vi "Acquisition Engine State Machine.vi"(5 "Start Next Record":bool, 7 "Record Parameters":T2={"Load Record Parameters?"=FALSE, "Pre Trigger Samples"=0, "Post Trigger Samples"=1000, "Trigger Hold Off"=0, "Record Count"=1}, 8 "Trigger Info":cluster{"Trigger":bool, "Trig Offset":u8}={"Trigger"=TRUE, "Trig Offset"=0}, 10 "Arm Acquisition Engine":bool, 11 "Input":i16[](array[numeric])=[0, 0, 0, 0, 0, 0, 0, 0]) -> (0 "Trigger Info":cluster{"Trigger":bool, "Trig Offset":u8}, 1 "PostTrigComplete":bool, 2 "AcqInProgress":bool, 3 "Output":i16[](array[numeric]), 4 "States":T1, 6 "Record Count":u32)   [LabVIEW 2012]
uses:
  <instrlib>/FlexRIO/Libraries/Acquisition Engine/FPGA/Interface/acqEngineStates v1.ctl
  <instrlib>/FlexRIO/Libraries/Acquisition Engine/FPGA/Implementation/acqEngineNRecordStateMachine.vi
  <vilib>/rvi/FXPMathLib/basic elements/FxpDiscreteDelay/XNode/nifxpmath_DiscreteDelay.xnode
  <instrlib>/FlexRIO/Libraries/Acquisition Engine/Acquisition Engine.lvlib
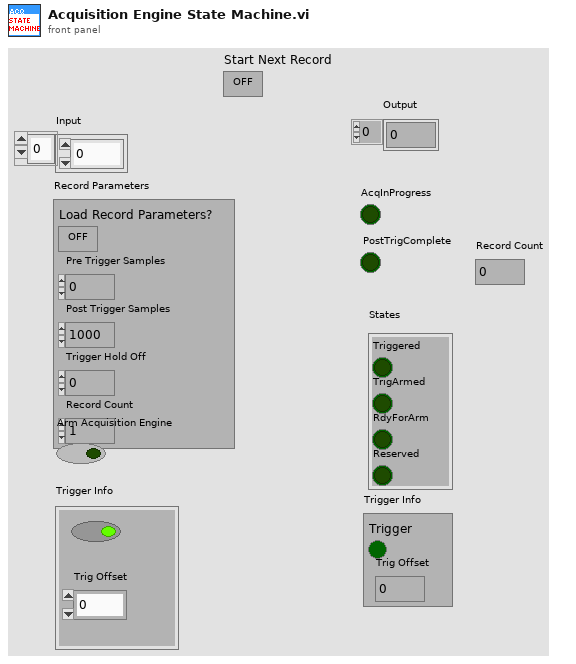
[diagram p1: front panel]
types:
  T1 = typedef "acqEngineStates v1.ctl" = cluster{"Triggered":bool, "TrigArmed":bool, "RdyForArm":bool, "Reserved":bool}
  T2 = cluster{"Load Record Parameters?":bool, "Pre Trigger Samples":u32, "Post Trigger Samples":u32, "Trigger Hold Off":u32, "Record Count":u32}
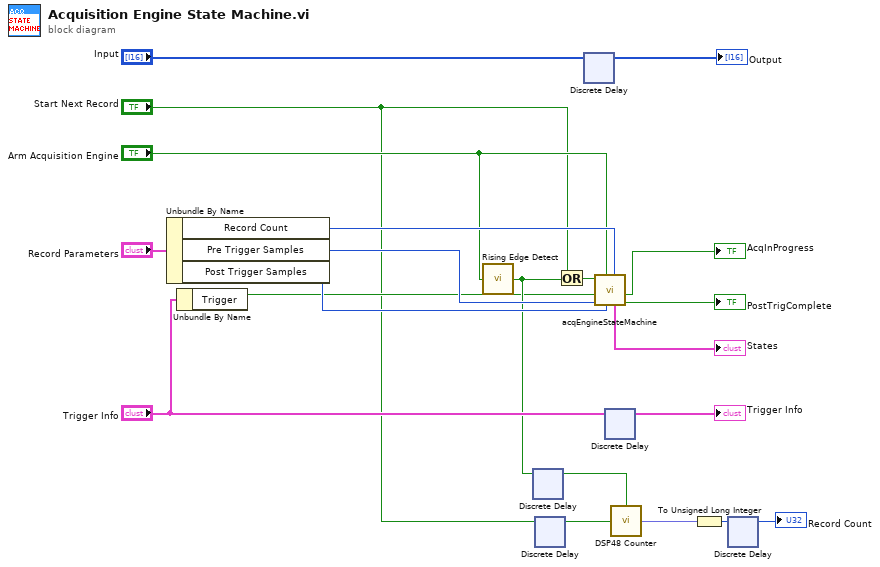
[diagram p0: block diagram]
diagram:
  n1 = Unbundle By Name("Record Parameters") -> ("Record Count"=w16:u32, "Pre Trigger Samples"=w17:u32, "Post Trigger Samples"=w18:u32)
  n2 = Unbundle By Name("Trigger Info") -> ("Trigger"=w7:bool)
  n3 = call <userlib>:"Rising Edge Detect.vi"("signal"="Arm Acquisition Engine") -> ("edge detected"=w8:bool)  [unwired: 14 in]
  n4 = xnode "Discrete Delay"("D"=w8) -> ("Q"=w3:bool)
  n5 = xnode "Discrete Delay"("D"="Start Next Record") -> ("Q"=w2:bool)
  n6 = Or(x="Start Next Record", y=w8) -> (x .or. y?=w21:bool)
  n7 = xnode "Discrete Delay"("D"="Input") -> ("Q"=→"Output":i16[])
  n8 = call-poly <instrlib>:"acqEngineStateMachine.vi"("acq.Record Count"=w16, "acq.Post Trig"=w18, "acq.Initiate"="Arm Acquisition Engine", "acq.Pre Trig"=w17, "Trig"=w7, "StartTrig"=w21) -> ("PostTrigComplete"=→"PostTrigComplete":bool, "AcqInProgress"=→"AcqInProgress":bool, "states"=→"States":T1)  [unwired: 3 in]
  n9 = xnode "Discrete Delay"("D"="Trigger Info") -> ("Q"=→"Trigger Info":cluster{"Trigger":bool, "Trig Offset":u8})
  n10 = call <userlib>:"DSP48 Counter.vi"("Reset ?"=w3, "Increment"=w2) -> ("Counter Value"=w1:fxp<+/-,48,48>)  [unwired: 12 in, 1 out]
  n11 = To Unsigned Long Integer(number=w1) -> (unsigned 32bit integer=w6:u32)
  n12 = xnode "Discrete Delay"("D"=w6) -> ("Q"=→"Record Count":u32)
